vi "TestWriteBlk.vi"() -> ()   [LabVIEW 2011]
panel:
  out "数值":i32
  out "偏移量（字节） 2":i64
  out "Image Pixels (U8)":u8[][][](array[numeric])
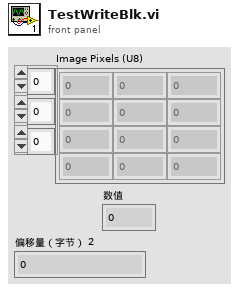
[diagram p1: front panel]
types:
  T1 = enum16{"big-endian, network order", "native, host order", "little-endian"}
  T2 = typedef "IMAQ Image.ctl" = refnum<image>
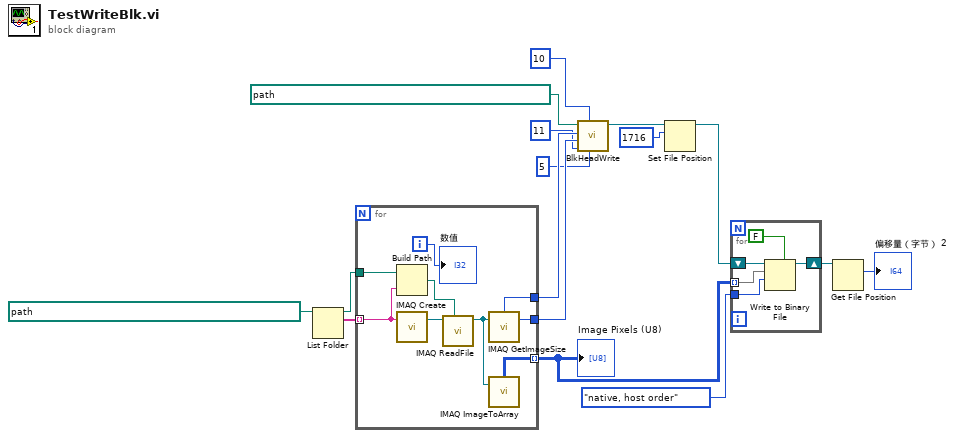
[diagram p0: block diagram]
diagram:
  n1 = List Folder(path=path "C:/Users/pan/Desktop/work/热成像/testimaging" ("路径")) -> (path out=w13:path, filenames=w14:string[])  [unwired: 3 in, 2 out]
  n2 = for {
    tunnel: w14 -> [w24] mode=indexing
    tunnel: w13 -> [w25]
    tunnel: [w21] -> w7 mode=indexing
    tunnel: [w19] -> w12
    tunnel: [w18] -> w11
    i -> [w17]
    n3 = Build Path(base path=w25, name or relative path=w24) -> (appended path=w23:path)
    n4 = call "IMAQ Create"("Image Name"=w24) -> ("New Image"=w22:T2)  [unwired: 4 in, 1 out]
    n5 = call "IMAQ ReadFile"("File Path"=w23, "Image"=w22) -> ("Image Out"=w20:T2)  [unwired: 5 in, 4 out]
    n6 = call "IMAQ GetImageSize"("Image"=w20) -> ("Y Resolution"=w18:i32, "X Resolution"=w19:i32)  [unwired: 3 in, 1 out]
    n7 = call "IMAQ ImageToArray"("Image"=w20) -> ("Image Pixels (U8)"=w21:u8[][])  [unwired: 3 in, 4 out]
    "数值" <- w17
  }
  "Image Pixels (U8)" <- w7
  n8 = call "BlkHeadWrite.vi"("Stimuli"=5, "FramesPerStim"=10, "datatype"=11, "FrameHeight"=w11, "FrameWidth"=w12, "BlkFilePath"=path "C:/Users/pan/Desktop/work/热成像/WriteTest.blk") -> ("引用句柄输出"=w2:refnum<file>)  [unwired: 5 in]
  n9 = Set File Position(offset (in bytes) (0)=i64 1716 ("偏移量（字节）（0）"), refnum=w2) -> (refnum out=w3:refnum<file>)  [unwired: 2 in, 1 out]
  n10 = for {
    tunnel: w7 -> [w29] mode=indexing
    shift-right: [w28] -> w6
    shift-left: w3 -> [w30]
    tunnel: T1."native, host order" ("字节顺序(0:big-endian, network order)") -> [w27]
    n11 = Write to Binary File(file (use dialog)=w30, data=w29, 5:FALSE ("预置数组或字符串大小？(T)"), 9:w27) -> (refnum out=w28:refnum<file>)  [unwired: 2 in, 2 out]
  }
  n12 = Get File Position(7:w6) -> (2:→"偏移量（字节） 2":i64)  [unwired: 1 in, 2 out]
